vi "Change Settings.vi"(8 "error in (no error)":errorcluster) -> (0 "error out":errorcluster)   [LabVIEW 2023]
doc: "Presents an interface to change any settings that have been established in the application."
uses:
  CTLs/Hotkey Type.ctl
  <vilib>/Utility/config.llb/Config Data RefNum.ctl
  CTLs/Hotkey Values.ctl
  CTLs/FGV Actions.ctl
  2b057859-5186-41e9-9ab4-790756e7a186.vi
  a5ac09e5-38d3-43bc-9feb-68748838b8f7.vi
  <vilib>/Utility/inputDevices.llb/closeKeyboard.vi
  <vilib>/Utility/inputDevices.llb/keyboardAcquire.vi
  FaKI State Machine/FaKI State Machine.lvlib
  <vilib>/Utility/config.llb/NI_LVConfig.lvlib
panel:
  in  "Hotkey Type":T1
  in  "Start/Stop":bool
  in  "Exit":bool
  # "Change Hotkey\nPress Start Listening and hold down a key combination for five seconds to assign it as a hotkey."
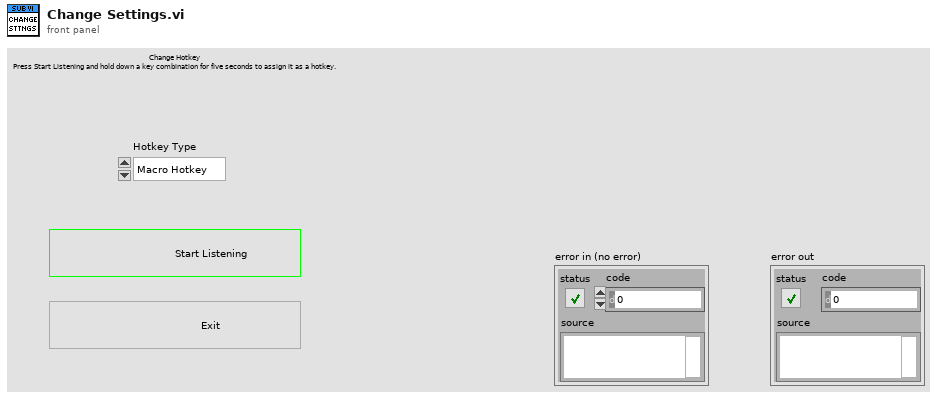
[diagram p1: front panel]
types:
  T1 = typedef "Hotkey Type.ctl" = enum16{"Macro Hotkey", "Abort Hotkey"}
  T2 = enum32{"Invalid", "Standard", "Closed", "Hidden", "Minimized", "Maximized"}
  T3 = enum32{"invalid app kind", "Development System", "Run Time System", "Student Edition", "Embedded LabVIEW", "Evaluation", "Custom"}
  T4 = typedef "FGV Actions.ctl" = enum16{"Read", "Write"}
  T5 = typedef "NI_LVConfig.lvlib/Config Data RefNum.ctl" = refnum<k1>
  T6 = typedef "Hotkey Values.ctl" = cluster{"Macro Hotkey":enum16{"0", "1", "2", "3", "4", "5", "6", "7", "8", "9", "A", "B", "C", "D", "E", "F", "G", "H", "I", "J", "K", "L", "M", "N", "O", "P", "Q", "R", "S", "T", "U", "V", "W", "X", "Y", "Z", "F1", "F2", "F3", "F4", "F5", "F6", "F7", "F8", "F9", "F10", "F11", "F12", "F13", "F14", "F15", "ADD", "BACK", "BACKSLASH", "CAPITAL", "COMMA", "DECIMAL", "DELETE", "DIVIDE", "DOWN", "END", "EQUALS", "ESCAPE", "GRAVE (`)", "HOME", "INSERT", "LBRACKET", "LCONTROL", "LEFT", "L ALT", "LSHIFT", "LWIN", "MINUS", "MULTIPLY", "NEXT", "NUMLOCK", "NUMPAD_0", "NUMPAD_1", "NUMPAD_2", "NUMPAD_3", "NUMPAD_4", "NUMPAD_5", "NUMPAD_6", "NUMPAD_7", "NUMPAD_8", "NUMPAD_9", "PAUSE", "PERIOD", "PRIOR (PG UP)", "RBRACKET", "RCONTROL", "RETURN", "RIGHT", "R ALT", "RSHIFT", "RWIN", "SCROLL", "SEMICOLON", "SLASH", "SPACE", "SUBTRACT", "TAB", "UP", "ENTER (num pad)", "' (quote)"}[], "Abort Hotkey":enum16{"0", "1", "2", "3", "4", "5", "6", "7", "8", "9", "A", "B", "C", "D", "E", "F", "G", "H", "I", "J", "K", "L", "M", "N", "O", "P", "Q", "R", "S", "T", "U", "V", "W", "X", "Y", "Z", "F1", "F2", "F3", "F4", "F5", "F6", "F7", "F8", "F9", "F10", "F11", "F12", "F13", "F14", "F15", "ADD", "BACK", "BACKSLASH", "CAPITAL", "COMMA", "DECIMAL", "DELETE", "DIVIDE", "DOWN", "END", "EQUALS", "ESCAPE", "GRAVE (`)", "HOME", "INSERT", "LBRACKET", "LCONTROL", "LEFT", "L ALT", "LSHIFT", "LWIN", "MINUS", "MULTIPLY", "NEXT", "NUMLOCK", "NUMPAD_0", "NUMPAD_1", "NUMPAD_2", "NUMPAD_3", "NUMPAD_4", "NUMPAD_5", "NUMPAD_6", "NUMPAD_7", "NUMPAD_8", "NUMPAD_9", "PAUSE", "PERIOD", "PRIOR (PG UP)", "RBRACKET", "RCONTROL", "RETURN", "RIGHT", "R ALT", "RSHIFT", "RWIN", "SCROLL", "SEMICOLON", "SLASH", "SPACE", "SUBTRACT", "TAB", "UP", "ENTER (num pad)", "' (quote)"}[]}
  T7 = cluster{"Core":cluster{"Current VI Reference":refnum<vi>, "Close Panel on Exit?":bool}, "Config":T5, "Keyboard":refnum<k1>, "Last":enum16{"0", "1", "2", "3", "4", "5", "6", "7", "8", "9", "A", "B", "C", "D", "E", "F", "G", "H", "I", "J", "K", "L", "M", "N", "O", "P", "Q", "R", "S", "T", "U", "V", "W", "X", "Y", "Z", "F1", "F2", "F3", "F4", "F5", "F6", "F7", "F8", "F9", "F10", "F11", "F12", "F13", "F14", "F15", "ADD", "BACK", "BACKSLASH", "CAPITAL", "COMMA", "DECIMAL", "DELETE", "DIVIDE", "DOWN", "END", "EQUALS", "ESCAPE", "GRAVE (`)", "HOME", "INSERT", "LBRACKET", "LCONTROL", "LEFT", "L ALT", "LSHIFT", "LWIN", "MINUS", "MULTIPLY", "NEXT", "NUMLOCK", "NUMPAD_0", "NUMPAD_1", "NUMPAD_2", "NUMPAD_3", "NUMPAD_4", "NUMPAD_5", "NUMPAD_6", "NUMPAD_7", "NUMPAD_8", "NUMPAD_9", "PAUSE", "PERIOD", "PRIOR (PG UP)", "RBRACKET", "RCONTROL", "RETURN", "RIGHT", "R ALT", "RSHIFT", "RWIN", "SCROLL", "SEMICOLON", "SLASH", "SPACE", "SUBTRACT", "TAB", "UP", "ENTER (num pad)", "' (quote)"}[], "Hotkeys":T6}
  T8 = enum16{"0", "1", "2", "3", "4", "5", "6", "7", "8", "9", "A", "B", "C", "D", "E", "F", "G", "H", "I", "J", "K", "L", "M", "N", "O", "P", "Q", "R", "S", "T", "U", "V", "W", "X", "Y", "Z", "F1", "F2", "F3", "F4", "F5", "F6", "F7", "F8", "F9", "F10", "F11", "F12", "F13", "F14", "F15", "ADD", "BACK", "BACKSLASH", "CAPITAL", "COMMA", "DECIMAL", "DELETE", "DIVIDE", "DOWN", "END", "EQUALS", "ESCAPE", "GRAVE (`)", "HOME", "INSERT", "LBRACKET", "LCONTROL", "LEFT", "L ALT", "LSHIFT", "LWIN", "MINUS", "MULTIPLY", "NEXT", "NUMLOCK", "NUMPAD_0", "NUMPAD_1", "NUMPAD_2", "NUMPAD_3", "NUMPAD_4", "NUMPAD_5", "NUMPAD_6", "NUMPAD_7", "NUMPAD_8", "NUMPAD_9", "PAUSE", "PERIOD", "PRIOR (PG UP)", "RBRACKET", "RCONTROL", "RETURN", "RIGHT", "R ALT", "RSHIFT", "RWIN", "SCROLL", "SEMICOLON", "SLASH", "SPACE", "SUBTRACT", "TAB", "UP", "ENTER (num pad)", "' (quote)"}[]
  T9 = cluster{"Current VI Reference":refnum<vi>, "Close Panel on Exit?":bool}
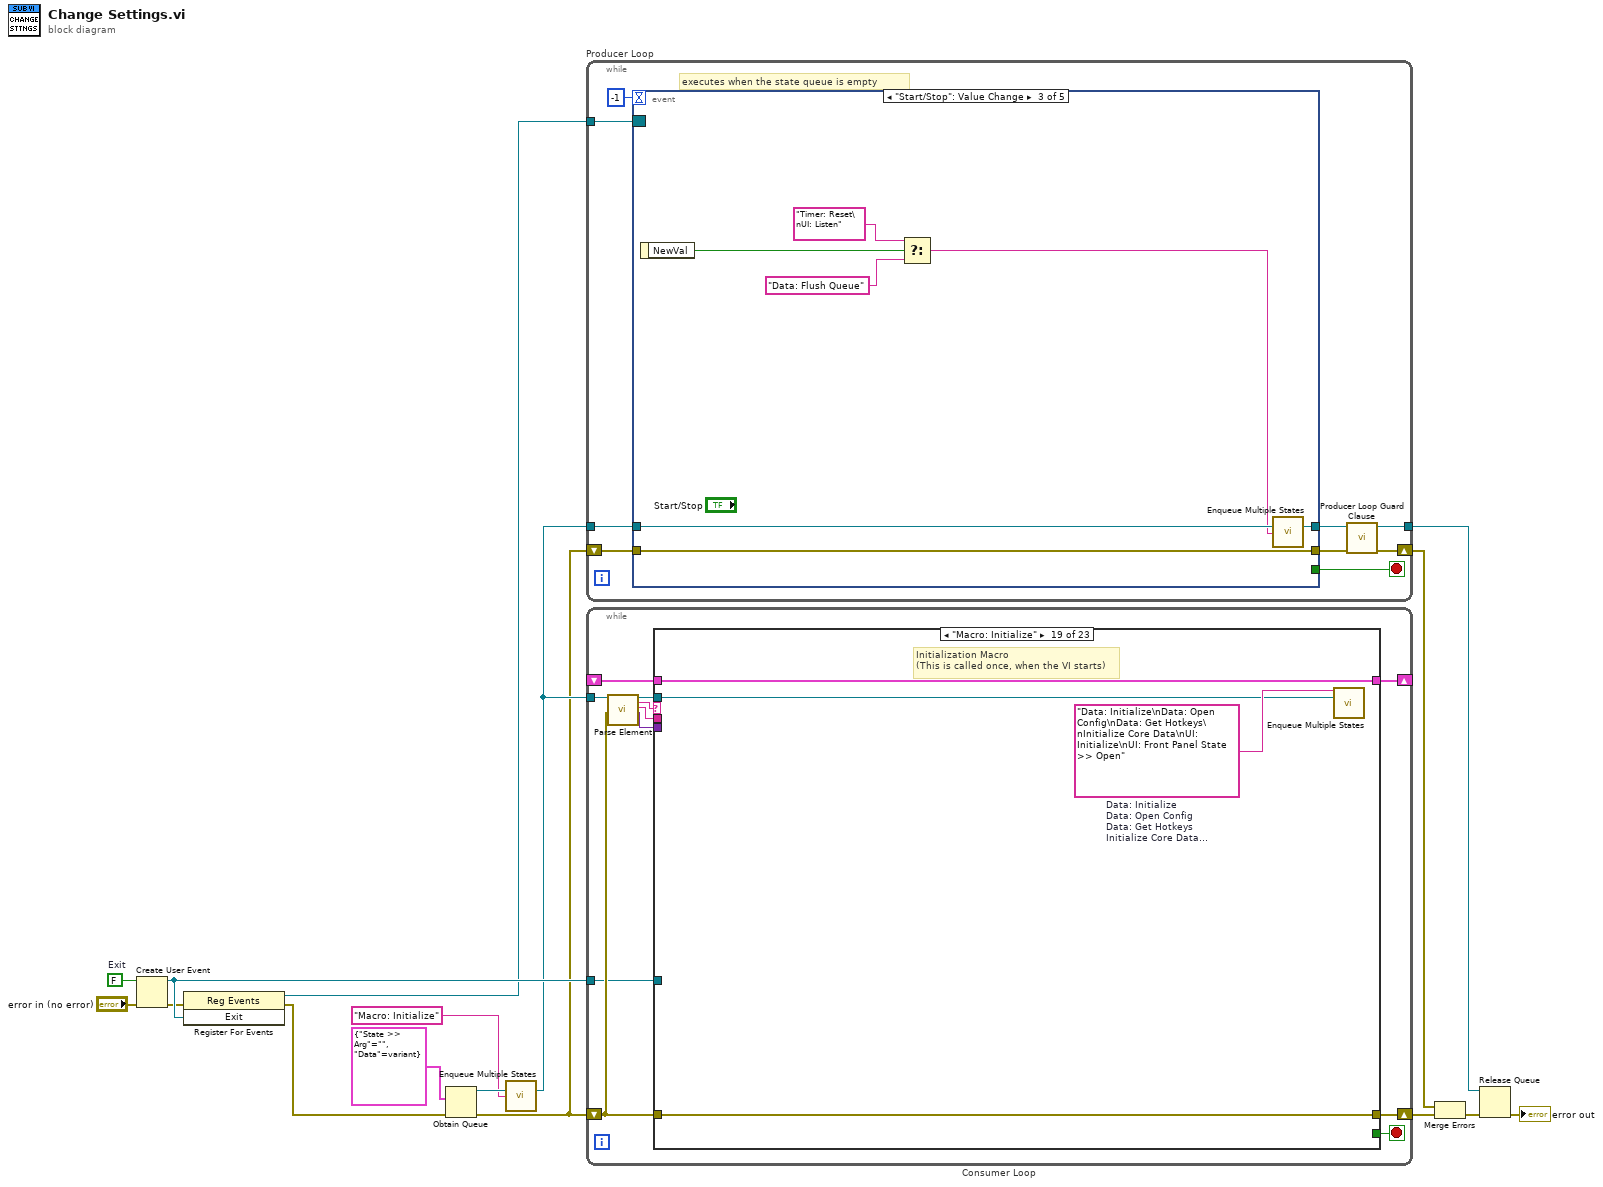
[diagram p0: block diagram]
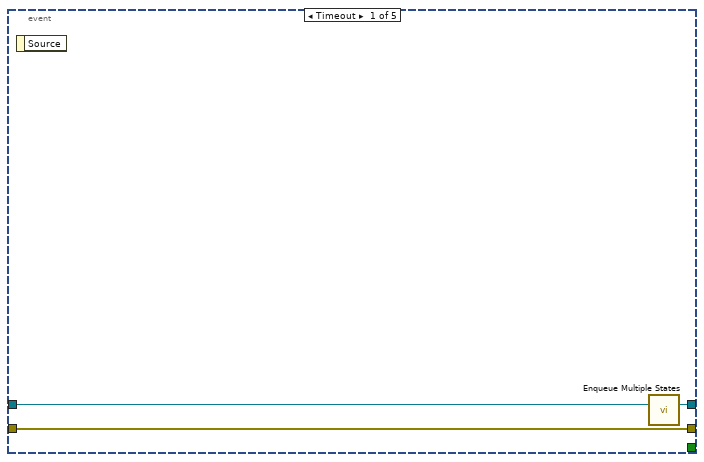
[diagram p2: hidden frame]
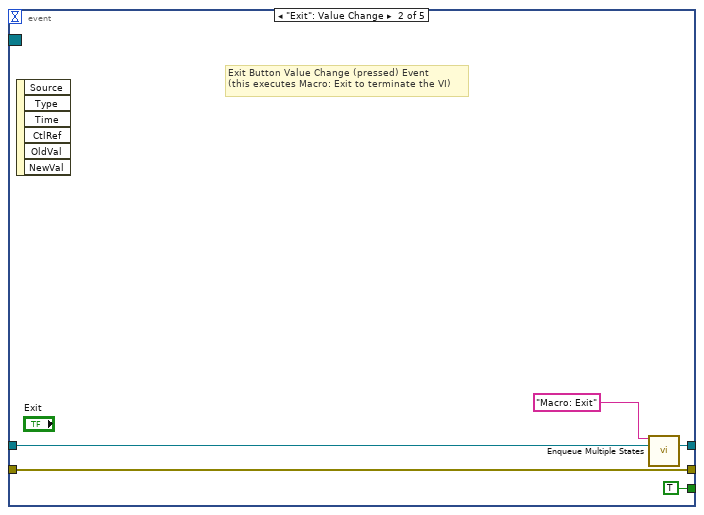
[diagram p3: hidden frame]
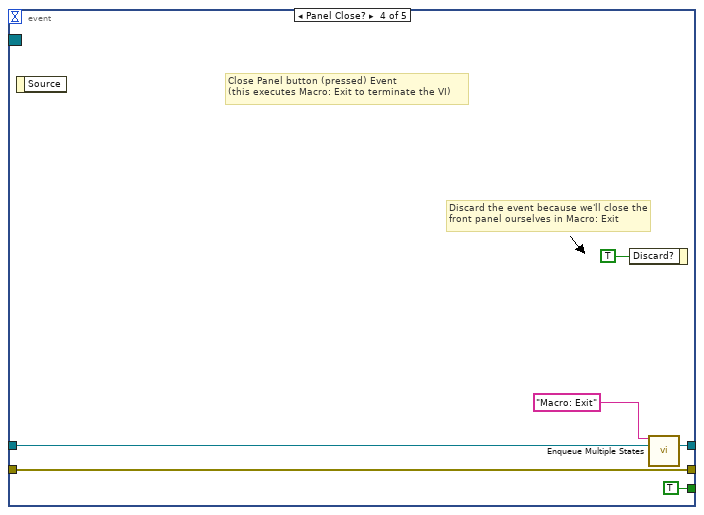
[diagram p4: hidden frame]
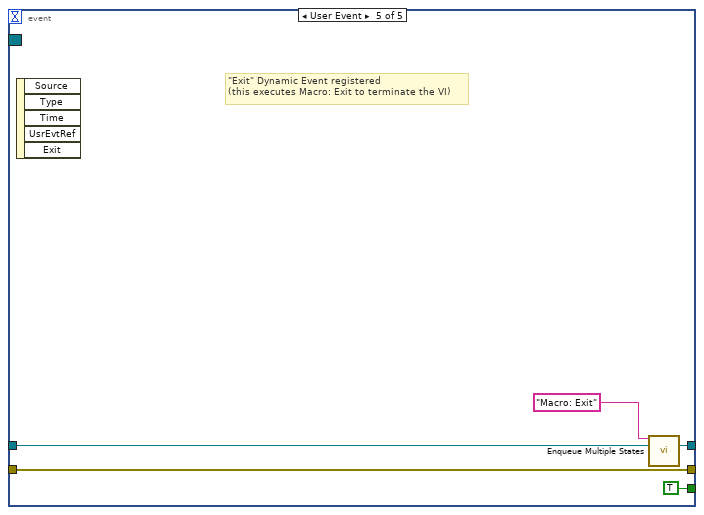
[diagram p5: hidden frame]
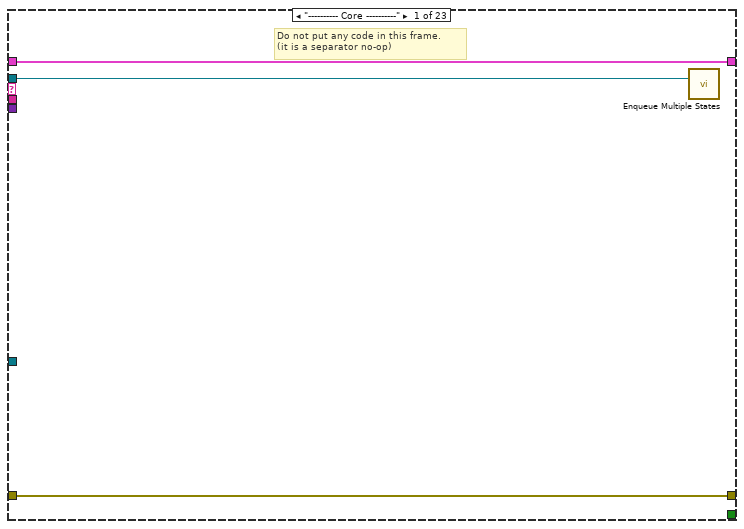
[diagram p6: hidden frame]
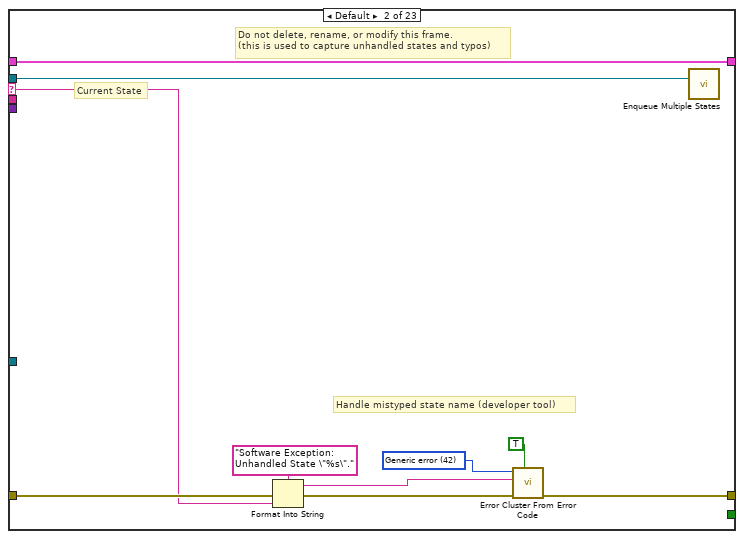
[diagram p7: hidden frame]
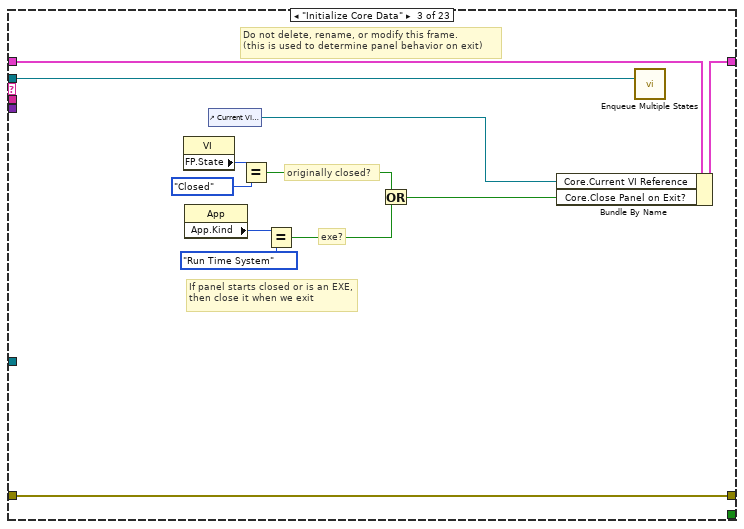
[diagram p8: hidden frame]
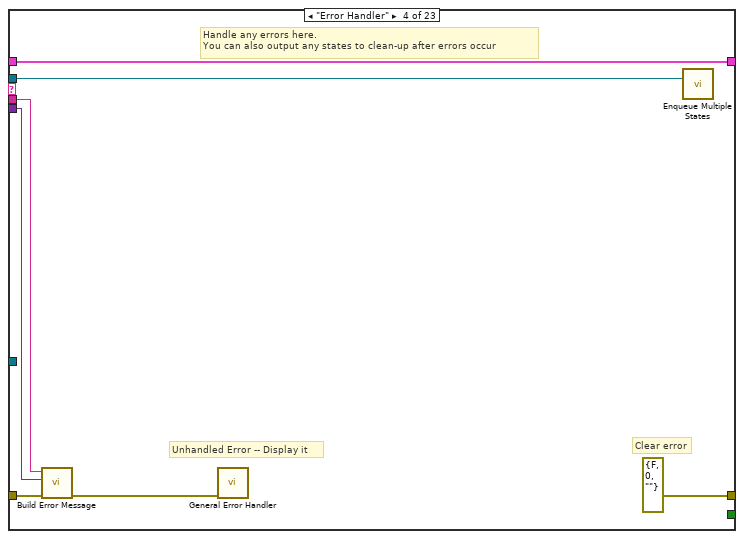
[diagram p9: hidden frame]
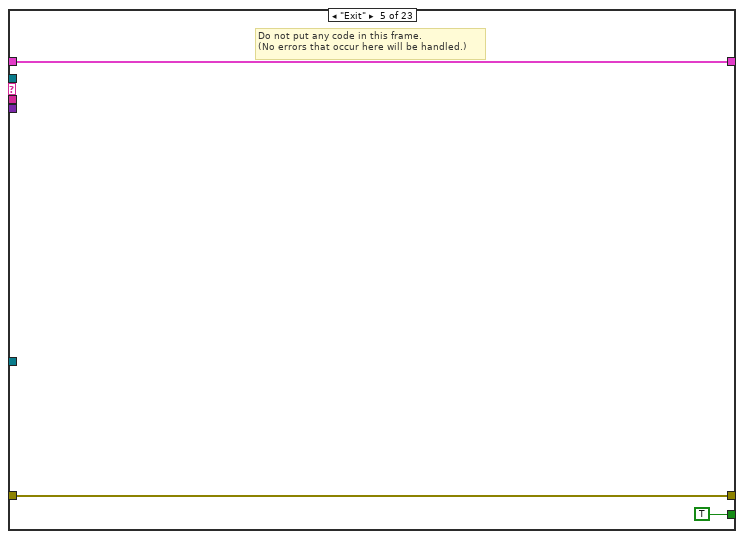
[diagram p10: hidden frame]
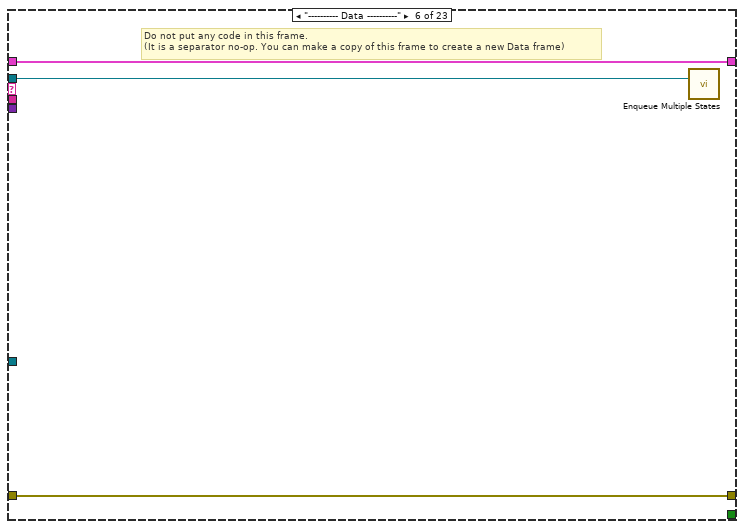
[diagram p11: hidden frame]
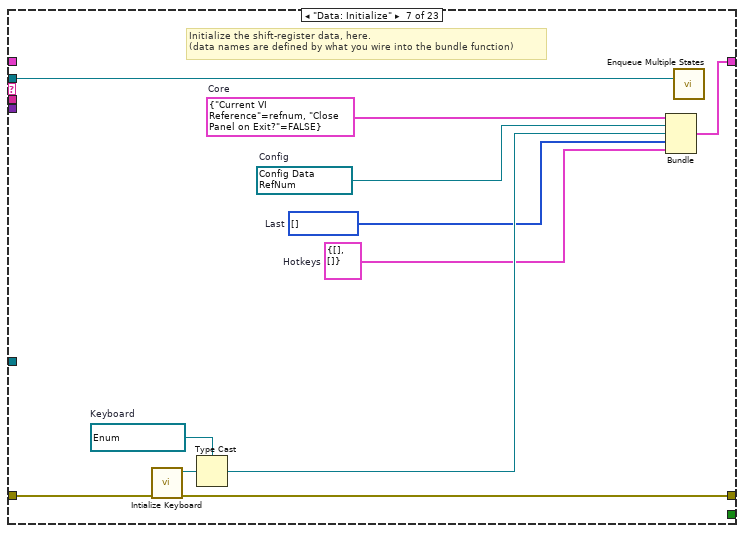
[diagram p12: hidden frame]
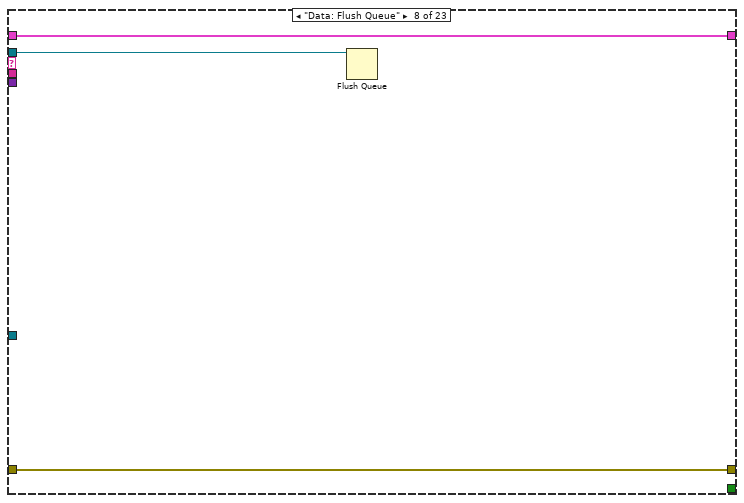
[diagram p13: hidden frame]
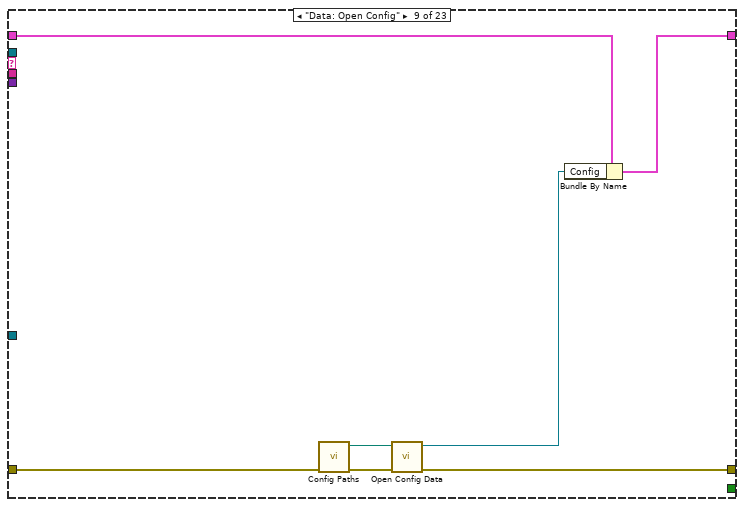
[diagram p14: hidden frame]
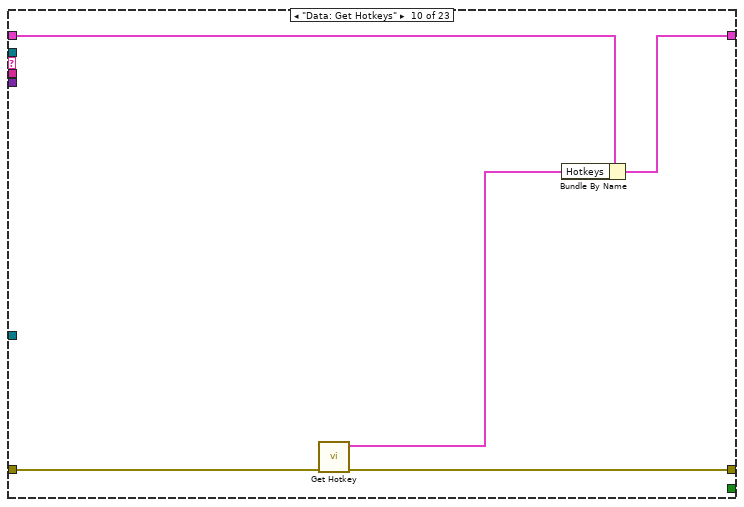
[diagram p15: hidden frame]
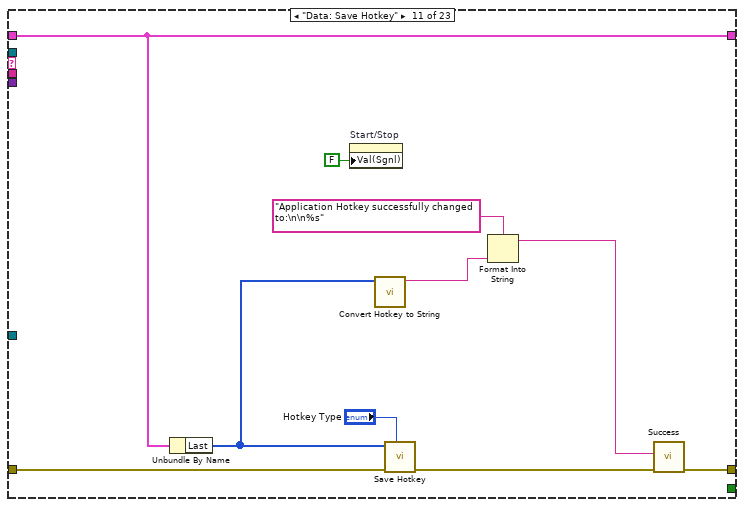
[diagram p16: hidden frame]
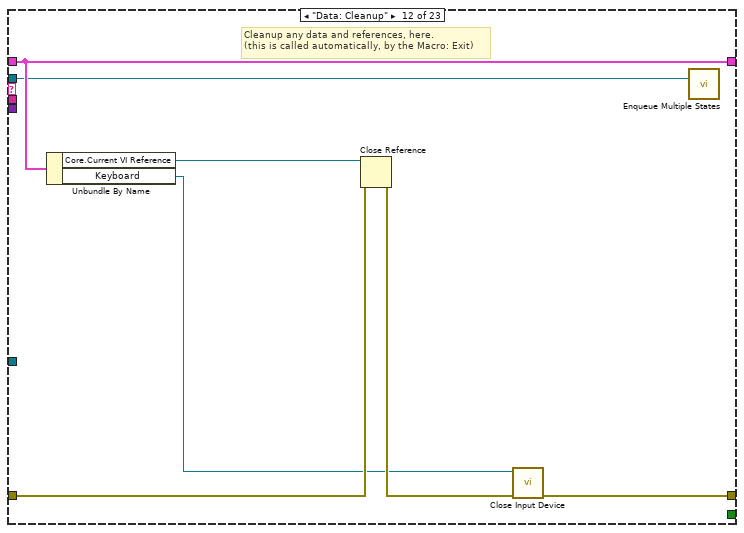
[diagram p17: hidden frame]
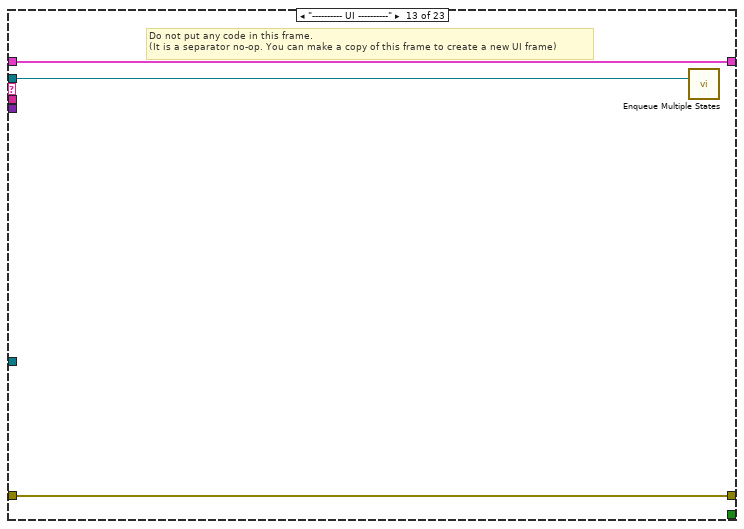
[diagram p18: hidden frame]
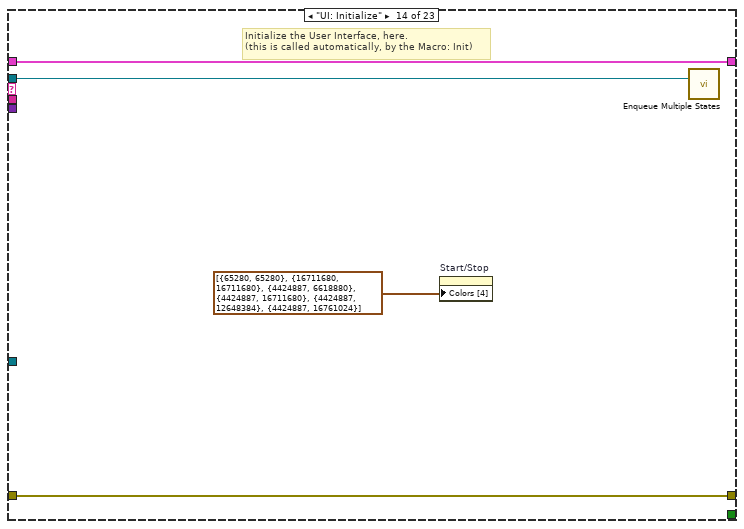
[diagram p19: hidden frame]
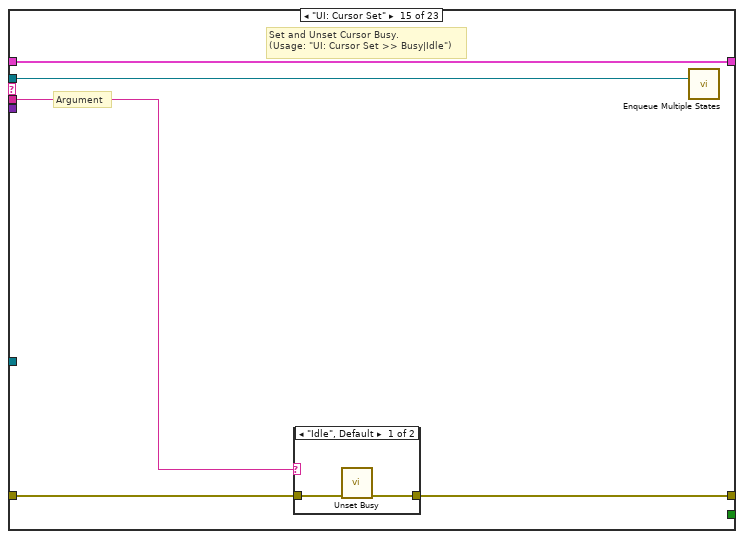
[diagram p20: hidden frame]
diagram:
  w13 = FALSE  # Exit
  n1 = Create User Event(user event datatype=w13, error in="error in (no error)") -> (user event=w16:refnum<user-event>, error out=w12:errorcluster)
  n2 = register-events(error in=w12, w16) -> (reference out=w15:refnum<event-registration>, error out=w14:errorcluster)  [unwired: 1 in]
  n3 = Obtain Queue(element data type=cluster{"State >> Arg":string, "Data":variant} {"State >> Arg"="", "Data"=variant}, error in (no error)=w14) -> (queue out=w6:refnum<queue>, error out=w3:errorcluster)  [unwired: 3 in, 1 out]
  n4 = call "Enqueue Multiple States.vi"("queue in"=w6, "State(s) at Back"="Macro: Initialize") -> ("queue out"=w7:refnum<queue>)  [unwired: 13 in]
  n5 = while "Producer Loop" {
    shift-right: [w20] -> w9
    shift-left: w3 -> [w25]
    tunnel: w15 -> [w17]
    tunnel: w7 -> [w23]
    tunnel: [w18] -> w11
    stop <- w22 stop-if-true
    # "executes when the state queue is empty"
    n6 = event shown="[2] \"Start/Stop\": Value Change" {
      selector: w17 -> [_ _ _ _ _]
      dyn-events: _ -> [_ _ _ _ _]
      timeout: -1 ("Timeout") -> [_ _ _ _ _]
      tunnel: [w26 w33 w40 w46 w51] -> w21
      tunnel: w25 -> [w26 w33 w40 w46 w51]
      tunnel: w23 -> [w27 w32 w39 w43 w49]
      tunnel: [w28 w30 w38 w42 w48] -> w19
      tunnel: [_ TRUE _ TRUE TRUE] -> w22
      event Timeout {
        n7 = event-data() -> ()  [unwired: 1 in, 1 out]
        n8 = call "Enqueue Multiple States.vi"("queue in"=w27) -> ("queue out"=w28:refnum<queue>)  [unwired: 14 in]
      }
      event "Exit": Value Change {
        # "Exit Button Value Change (pressed) Event\n(this executes Macro: Exit to terminate the VI)"
        n9 = event-data() -> ()  [unwired: 1 in, 6 out]
        n10 = call "Enqueue Multiple States.vi"("State(s) at Front"="Macro: Exit", "queue in"=w32) -> ("queue out"=w30:refnum<queue>)  [unwired: 13 in]
      }
      event "Start/Stop": Value Change {
        n11 = event-data() -> ("NewVal"=w37:bool)  [unwired: 1 in]
        n12 = Select(t="Timer: Reset\nUI: Listen", s=w37, f="Data: Flush Queue") -> (s? t:f=w34:string)
        n13 = call "Enqueue Multiple States.vi"("queue in"=w39, "State(s) at Back"=w34) -> ("queue out"=w38:refnum<queue>)  [unwired: 13 in]
      }
      event Panel Close? {
        # "Discard the event because we'll close the front panel ourselves in Macro: Exit"
        # "Close Panel button (pressed) Event\n(this executes Macro: Exit to terminate the VI)"
        n14 = event-data() -> ()  [unwired: 1 in, 1 out]
        n15 = event-data("Discard?"=TRUE) -> ()  [unwired: 1 in, 1 out]
        n16 = call "Enqueue Multiple States.vi"("State(s) at Front"="Macro: Exit", "queue in"=w43) -> ("queue out"=w42:refnum<queue>)  [unwired: 13 in]
      }
      event User Event {
        # "\"Exit\" Dynamic Event registered\n(this executes Macro: Exit to terminate the VI)"
        n17 = event-data() -> ()  [unwired: 1 in, 5 out]
        n18 = call "Enqueue Multiple States.vi"("State(s) at Front"="Macro: Exit", "queue in"=w49) -> ("queue out"=w48:refnum<queue>)  [unwired: 13 in]
      }
    }
    n19 = call "Producer Loop Guard Clause.vi"("error in (no error)"=w21, "queue in"=w19) -> ("error out"=w20:errorcluster, "queue out"=w18:refnum<queue>)  [unwired: 8 in]
  }
  n20 = while "Consumer Loop" {
    shift-right: [w59] -> _
    shift-left: _ -> [w58]
    shift-right: [w62] -> w8
    shift-left: w3 -> [w61]
    tunnel: w7 -> [w57]
    tunnel: w16 -> [w52]
    stop <- w60 stop-if-true
    n21 = call "Parse Element.vi"("queue in"=w57, "error in (no error)"=w61) -> ("queue out"=w56:refnum<queue>, "State"=w55:string, "Arg"=w54:string, "Data"=w53:variant)  [unwired: 14 in]
    n22 = case shown="\"Macro: Initialize\"" w55 {
      selector: w55 -> [_ w67 _ _ _ _ _ _ _ _ _ _ _ _ _ _ _ _ _ _ _ _ _]
      tunnel: w56 -> [w63 w66 w76 w92 _ w98 w109 w114 _ _ _ w140 w144 w148 w151 w160 w243 w266 w269 w276 w282 _ w291]
      tunnel: w54 -> [_ _ _ w88 _ _ _ _ _ _ _ _ _ _ w152 w161 _ _ _ _ _ _ _]
      tunnel: w58 -> [w64 w69 w82 w93 w96 w99 _ w113 w118 w125 w127 w141 w145 w149 w153 w163 w242 w267 w271 w280 w283 w289 w298]
      tunnel: [w65 w74 w87 errorcluster {"status"=FALSE, "code"=0, "source"=""} ("error out") w97 w100 w103 w112 w119 w123 w134 w138 w146 w150 w154 w164 w251 w268 w272 w281 w284 w287 w296] -> w62
      tunnel: w61 -> [w65 w73 w87 w91 w97 w100 w106 w112 w120 w126 w132 w143 w146 w150 w155 w165 w252 w268 w272 w281 w284 w288 w297]
      tunnel: [_ _ _ _ TRUE _ _ _ _ _ _ _ _ _ _ _ _ _ _ _ _ _ _] -> w60
      tunnel: [w64 w69 w86 w93 w96 w99 w111 w113 w117 w124 w127 w141 w145 w149 w153 w163 w241 w267 w271 w280 w283 w289 w298] -> w59
      tunnel: w53 -> [_ _ _ w89 _ _ _ _ _ _ _ _ _ _ _ _ _ _ _ _ _ _ _]
      tunnel: w52 -> [_ _ _ _ _ _ _ _ _ _ _ _ _ _ _ _ _ _ _ _ _ _ _]
      frame "---------- Core ----------" {
        # "Do not put any code in this frame.\n(it is a separator no-op)"
        n23 = call "Enqueue Multiple States.vi"("queue in"=w63) -> ()  [unwired: 14 in, 1 out]
      }
      frame Default {
        w71 = 42 items=["No error", "Argument error", "Memory is full", "Out of zone", "End of file", "File already open", "Generic file I/O error", "File not found", "File permission error", "Disk is full", "Duplicate path", "Too many files open", "System feature not enabled", "Resource file not found", "Cannot add resource", "Resource not found", "Image not found", "Image memory error", "Pen does not exist", "Config type invalid", "Config token not found", "Config parse error", "Config memory error", "Bad external code format", "Bad external code offset", "External code not present", "Null window", "Destroy window error", "Null menu", "Print aborted", "Bad print record", "Print driver error", "Windows error during printing", "Memory error during printing", "Print dialog error", "Generic print error", "Invalid device refnum", "Device not found", "Device parameter error", "Device unit error", "Cannot open device", "Device call aborted", "Generic error", "Cancelled by user", "Object ID too low", "Object ID too high", "Object not in heap", "Unknown heap", "Unknown object (invalid DefProc)", "Unknown object (DefProc not in table)", "Message out of range", "Invalid (null) method", "Unknown message", "Manager call not supported", "Bad address", "Network operation in progress", "Network operation timed out", "Connection is busy", "Network attribute not supported", "Network error", "Address in use", "System out of memory", "Connection aborted", "Connection refused", "Not connected", "Already connected", "Connection closed", "Initialization error (interapplication manager)", "Bad occurrence", "Wait on unbound occurrence handler", "Occurrence queue overflow", "Datalog type conflict", "Unused", "Unrecognized type (interapplication manager)", "Memory corrupt", "Failed to make temporary DLL", "Old CIN version", "Drag socket not found", "Failed to load drop-object", "Failed to register OLE object", "Failed to release OLE object", "Format specifier type mismatch", "Unknown format specifier", "Too few format specifiers", "Too many format specifiers", "Scan failed", "Newer CIN version", "Error converting to variant", "Runtime menu error", "Password tampered", "Variant attribute not found", "Incompatible variant data type", "Event data is not available", "Event Store is not present", "Occurrence is not found", "Event Queue is not created", "Event info is not available", "Refnum passed is NULL", "Error retrieving Class GUID", "Error retrieving CoClass GUID", "Error retrieving TypeLib GUID.", "Bad built application magic bytes.", "Specific driver is different from the specific driver associated with the Logical Name.", "There is no session opened to the class driver.", "Max Error", "MAX - Error with config objects", "MAX - Error loading configuration", "MAX - Group not supported"]
        # "Current State"
        # "Do not delete, rename, or modify this frame.\n(this is used to capture unhandled states and typos)"
        # "Handle mistyped state name (developer tool)"
        n24 = Format Into String(format string="Software Exception: Unhandled State \"%s\"." ("message"), error in=w73, w67) -> (resulting string=w70:string, error out=w75:errorcluster)  [unwired: 1 in]
        n25 = call <vilib>:"Error Cluster From Error Code.vi"("show call chain? (False)"=TRUE, "error in (no error)"=w75, "error message (\"\")"=w70, "error code (0)"=w71) -> ("error out"=w74:errorcluster)  [unwired: 5 in]
        n26 = call "Enqueue Multiple States.vi"("queue in"=w66) -> ()  [unwired: 14 in, 1 out]
      }
      frame "Initialize Core Data" {
        # "Do not delete, rename, or modify this frame.\n(this is used to determine panel behavior on exit)"
        # "originally closed?"
        # "exe?"
        # "If panel starts closed or is an EXE, then close it when we exit"
        n27 = property class="VI"() -> ("FP.State"=w79:T2)  [unwired: 2 in, 2 out]
        n28 = property class="App"() -> ("App.Kind"=w85:T3)  [unwired: 2 in, 2 out]
        n29 = control-ref of="Current VI Reference"() -> (w80:refnum<vi>)
        n30 = Equal?(x=w79, y=T2."Closed" ("Front Panel Window:State")) -> (x = y?=w77:bool)
        n31 = Equal?(x=w85, y=T3."Run Time System" ("Application:Kind")) -> (x = y?=w83:bool)
        n32 = Or(x=w77, y=w83) -> (x .or. y?=w81:bool)
        n33 = Bundle By Name(cluster=w82, "Core.Current VI Reference"=w80, "Core.Close Panel on Exit?"=w81) -> (w86:T7)
        n34 = call "Enqueue Multiple States.vi"("queue in"=w76) -> ()  [unwired: 14 in, 1 out]
      }
      frame "Error Handler" {
        # "Unhandled Error -- Display it"
        # "Handle any errors here.\nYou can also output any states to clean-up after errors occur"
        # "Clear error"
        n35 = call "Build Error Message.vi"("error in (no error)"=w91, "Data"=w89, "Arg"=w88) -> ("error out"=w90:errorcluster)  [unwired: 8 in]
        n36 = call <vilib>:"General Error Handler.vi"("error in (no error)"=w90) -> ()  [unwired: 10 in, 5 out]
        n37 = call "Enqueue Multiple States.vi"("queue in"=w92) -> ()  [unwired: 14 in, 1 out]
      }
      frame "Exit" {
        # "Do not put any code in this frame.\n(No errors that occur here will be handled.)"
      }
      frame "---------- Data ----------" {
        # "Do not put any code in this frame.\n(It is a separator no-op. You can make a copy of this frame to create a new Data frame)"
        n38 = call "Enqueue Multiple States.vi"("queue in"=w98) -> ()  [unwired: 14 in, 1 out]
      }
      frame "Data: Initialize" {
        w101 = T6 {"Macro Hotkey"=[], "Abort Hotkey"=[]}  # Hotkeys
        w102 = T8 [] items=["0", "1", "2", "3", "4", "5", "6", "7", "8", "9", "A", "B", "C", "D", "E", "F", "G", "H", "I", "J", "K", "L", "M", "N", "O", "P", "Q", "R", "S", "T", "U", "V", "W", "X", "Y", "Z", "F1", "F2", "F3", "F4", "F5", "F6", "F7", "F8", "F9", "F10", "F11", "F12", "F13", "F14", "F15", "ADD", "BACK", "BACKSLASH", "CAPITAL", "COMMA", "DECIMAL", "DELETE", "DIVIDE", "DOWN", "END", "EQUALS", "ESCAPE", "GRAVE (`)", "HOME", "INSERT", "LBRACKET", "LCONTROL", "LEFT", "L ALT", "LSHIFT", "LWIN", "MINUS", "MULTIPLY", "NEXT", "NUMLOCK", "NUMPAD_0", "NUMPAD_1", "NUMPAD_2", "NUMPAD_3", "NUMPAD_4", "NUMPAD_5", "NUMPAD_6", "NUMPAD_7", "NUMPAD_8", "NUMPAD_9", "PAUSE", "PERIOD", "PRIOR (PG UP)", "RBRACKET", "RCONTROL", "RETURN", "RIGHT", "R ALT", "RSHIFT", "RWIN", "SCROLL", "SEMICOLON", "SLASH", "SPACE", "SUBTRACT", "TAB", "UP", "ENTER (num pad)", "' (quote)"]  # Last
        w105 = T5 refnum items=["config data"]  # Config
        w107 = refnum<k1> refnum items=["KEYBOARD"]  # Keyboard
        w110 = T9 {"Current VI Reference"=refnum, "Close Panel on Exit?"=FALSE}  # Core
        # "Initialize the shift-register data, here.\n(data names are defined by what you wire into the bundle function)"
        n39 = call <vilib>:"Intialize Keyboard.vi"("error in (no error)"=w106) -> ("error out"=w103:errorcluster, "device ID"=w108:refnum<k1>)  [unwired: 9 in]
        n40 = Type Cast(type=w107, x=w108) -> (*(type *) &x=w104:refnum<k1>)
        n41 = Bundle("Core"=w110, "Config"=w105, "Keyboard"=w104, "Last"=w102, "Hotkeys"=w101) -> (w111:T7)  [unwired: 1 in]
        n42 = call "Enqueue Multiple States.vi"("queue in"=w109) -> ()  [unwired: 14 in, 1 out]
      }
      frame "Data: Flush Queue" {
        n43 = Flush Queue(queue=w114) -> ()  [unwired: 1 in, 3 out]
      }
      frame "Data: Open Config" {
        n44 = call "Config Paths.vi"("error in (no error)"=w120) -> ("error out"=w121:errorcluster, "Global Config"=w115:path)  [unwired: 8 in, 1 out]
        n45 = call <vilib>:"Open Config Data.vi"("error in (no error)"=w121, "configuration file path"=w115) -> ("error out"=w119:errorcluster, "refnum"=w116:T5)  [unwired: 7 in, 1 out]
        n46 = Bundle By Name(cluster=w118, "Config"=w116) -> (w117:T7)
      }
      frame "Data: Get Hotkeys" {
        n47 = call "Get Hotkey.vi"("error in (no error)"=w126) -> ("error out"=w123:errorcluster, "Hotkey Values"=w122:T6)  [unwired: 9 in]
        n48 = Bundle By Name(cluster=w125, "Hotkeys"=w122) -> (w124:T7)
      }
      frame "Data: Save Hotkey" {
        n49 = Unbundle By Name(w127) -> ("Last"=w129:T8)
        n50 = property on="Start/Stop" class="Bool (strict)"("Val(Sgnl)"=FALSE ("Value (Signaling)")) -> ()  [unwired: 2 in, 2 out]
        n51 = call "Convert Hotkey to String.vi"("Hotkey"=w129) -> ("String"=w128:string)  [unwired: 10 in]
        n52 = call "Save Hotkey.vi"("Hotkey Type"="Hotkey Type", "error in (no error)"=w132, "Hotkey"=w129) -> ("error out"=w131:errorcluster)  [unwired: 8 in]
        n53 = Format Into String(format string="Application Hotkey successfully changed to:\n\n%s", w128) -> (resulting string=w135:string)  [unwired: 2 in, 1 out]
        n54 = call "Success"("error in (no error)"=w131, "Message"=w135) -> ("error out"=w134:errorcluster)  [unwired: 8 in, 1 out]
      }
      frame "Data: Cleanup" {
        # "Cleanup any data and references, here.\n(this is called automatically, by the Macro: Exit)"
        n55 = Unbundle By Name(w141) -> ("Core.Current VI Reference"=w142:refnum<vi>, "Keyboard"=w137:refnum<k1>)
        n56 = Close Reference(reference=w142, error in (no error)=w143) -> (error out=w139:errorcluster)
        n57 = call-poly <vilib>:"Close Input Device.vi"("error in (no error)"=w139, "device ID"=w137) -> ("error out"=w138:errorcluster)  [unwired: 8 in]
        n58 = call "Enqueue Multiple States.vi"("queue in"=w140) -> ()  [unwired: 14 in, 1 out]
      }
      frame "---------- UI ----------" {
        # "Do not put any code in this frame.\n(It is a separator no-op. You can make a copy of this frame to create a new UI frame)"
        n59 = call "Enqueue Multiple States.vi"("queue in"=w144) -> ()  [unwired: 14 in, 1 out]
      }
      frame "UI: Initialize" {
        # "Initialize the User Interface, here.\n(this is called automatically, by the Macro: Init)"
        n60 = property on="Start/Stop" class="Bool (strict)"("Colors [4]"=cluster{u32, u32}[] [{65280, 65280}, {16711680, 16711680}, {4424887, 6618880}, {4424887, 16711680}, {4424887, 12648384}, {4424887, 16761024}]) -> ()  [unwired: 2 in, 2 out]
        n61 = call "Enqueue Multiple States.vi"("queue in"=w148) -> ()  [unwired: 14 in, 1 out]
      }
      frame "UI: Cursor Set" {
        # "Argument"
        # "Set and Unset Cursor Busy.\n(Usage: \"UI: Cursor Set >> Busy|Idle\")"
        n62 = case shown="\"Idle\", Default" w152 {
          tunnel: w155 -> [w157 w159]
          tunnel: [w156 w158] -> w154
          frame "Idle", Default {
            n63 = call <vilib>:"Unset Busy.vi"("error in (no error)"=w157) -> ("error out"=w156:errorcluster)  [unwired: 10 in]
          }
          frame "Busy" {
            n64 = call <vilib>:"Set Busy.vi"("error in (no error)"=w159) -> ("error out"=w158:errorcluster)  [unwired: 9 in, 1 out]
          }
        }
        n65 = call "Enqueue Multiple States.vi"("queue in"=w151) -> ()  [unwired: 14 in, 1 out]
      }
      frame "UI: Front Panel State" {
        # "Argument"
        # "Set Front Panel Open or Closed\n(Usage: \"UI: Front Panel State >> Open|Close\")"
        n66 = Unbundle By Name(w163) -> ("Core.Current VI Reference"=w162:refnum<vi>)
        n67 = case shown="\"Open\", \"Standard\", Default" w161 {
          tunnel: w165 -> [w172 w186 w198 w211 w224]
          tunnel: [w173 w187 w199 w212 w225] -> w164
          tunnel: w162 -> [w170 w184 w196 w209 w222]
          frame "Open", "Standard", Default {
            w166 = T2."Standard" ("State")
            n68 = property class="VI"(reference=w170, error in=w172) -> (reference out=w169:refnum<vi>, error out=w171:errorcluster, "FP.State"=w168:T2)
            n69 = Not Equal?(x=w168, y=w166) -> (x != y?=w167:bool)
            n70 = case shown="True" w167 {
              tunnel: [w178 w179] -> w173
              tunnel: w171 -> [w177 w179]
              tunnel: w169 -> [w175 _]
              tunnel: w166 -> [w174 _]
              frame True {
                n71 = invoke class="VI" method="FP.Open"(reference=w175, error in=w177, "Activate"=TRUE, "State"=w174) -> (error out=w178:errorcluster)  [unwired: 1 in, 4 out]
              }
              frame False {
              }
            }
          }
          frame "Close", "Closed" {
            n72 = property class="VI"(reference=w184, error in=w186) -> (reference out=w183:refnum<vi>, error out=w185:errorcluster, "FP.State"=w181:T2)
            n73 = Not Equal?(x=w181, y=T2."Closed" ("Front Panel Window:State")) -> (x != y?=w180:bool)
            n74 = case shown="True" w180 {
              tunnel: [w188 w191] -> w187
              tunnel: w185 -> [w188 w190]
              tunnel: w183 -> [_ w189]
              frame False {
              }
              frame True {
                n75 = invoke class="VI" method="FP.Close"(reference=w189, error in=w190) -> (error out=w191:errorcluster)  [unwired: 1 in, 2 out]
              }
            }
          }
          frame "Hidden", "Hide" {
            w192 = T2."Hidden" ("State")
            n76 = property class="VI"(reference=w196, error in=w198) -> (reference out=w195:refnum<vi>, error out=w197:errorcluster, "FP.State"=w194:T2)
            n77 = Not Equal?(x=w194, y=w192) -> (x != y?=w193:bool)
            n78 = case shown="True" w193 {
              tunnel: [w203 w204] -> w199
              tunnel: w197 -> [w202 w204]
              tunnel: w195 -> [w201 _]
              tunnel: w192 -> [w200 _]
              frame True {
                n79 = invoke class="VI" method="FP.Open"(reference=w201, error in=w202, "State"=w200) -> (error out=w203:errorcluster)  [unwired: 2 in, 4 out]
              }
              frame False {
              }
            }
          }
          frame "Minimize", "Minimized" {
            w205 = T2."Minimized" ("State")
            n80 = property class="VI"(reference=w209, error in=w211) -> (reference out=w208:refnum<vi>, error out=w210:errorcluster, "FP.State"=w207:T2)
            n81 = Not Equal?(x=w207, y=w205) -> (x != y?=w206:bool)
            n82 = case shown="True" w206 {
              tunnel: [w216 w217] -> w212
              tunnel: w210 -> [w215 w217]
              tunnel: w208 -> [w214 _]
              tunnel: w205 -> [w213 _]
              frame True {
                n83 = invoke class="VI" method="FP.Open"(reference=w214, error in=w215, "State"=w213) -> (error out=w216:errorcluster)  [unwired: 2 in, 4 out]
              }
              frame False {
              }
            }
          }
          frame "Maximize", "Maximized" {
            w218 = T2."Maximized" ("State")
            n84 = property class="VI"(reference=w222, error in=w224) -> (reference out=w221:refnum<vi>, error out=w223:errorcluster, "FP.State"=w220:T2)
            n85 = Not Equal?(x=w220, y=w218) -> (x != y?=w219:bool)
            n86 = case shown="True" w219 {
              tunnel: [w229 w230] -> w225
              tunnel: w223 -> [w228 w230]
              tunnel: w221 -> [w227 _]
              tunnel: w218 -> [w226 _]
              frame True {
                n87 = invoke class="VI" method="FP.Open"(reference=w227, error in=w228, "State"=w226) -> (error out=w229:errorcluster)  [unwired: 2 in, 4 out]
              }
              frame False {
              }
            }
          }
        }
        n88 = call "Enqueue Multiple States.vi"("queue in"=w160) -> ()  [unwired: 14 in, 1 out]
      }
      frame "UI: Listen" {
        n89 = Unbundle By Name(w242) -> ("Hotkeys"=w237:T6, "Last"=w249:T8, "Keyboard"=w256:refnum<k1>)
        n90 = call "Stall Data Flow.vim"("value in"=w256, "milliseconds to wait"=u32 1) -> ("value out"=w254:refnum<k1>)  [unwired: 1 out]
        n91 = Empty Array?(array=w249) -> (empty?=w250:bool)
        n92 = call-poly <vilib>:"Acquire Input Data.vi"("device ID"=w254, "error in (no error)"=w252) -> ("keys pressed"=w255:T8, "error out"=w251:errorcluster)  [unwired: 15 in, 1 out]
        n93 = call "Enum to Array of Enums.vim"("enum"=Hotkey_Type."Macro Hotkey" ("Hotkey Type")) -> ("array of enums"=w239:T1[])
        n94 = Not(x=w250) -> (.not. x?=w247:bool)
        n95 = Sort 1D Array(array=w255) -> (sorted array=w236:T8)
        n96 = Equal?(x=w249, y=w236) -> (x = y?=w248:bool)
        n97 = for {
          tunnel: w239 -> [w260] mode=indexing
          tunnel: w237 -> [w261]
          tunnel: [w260] -> w234 if=w257
          tunnel: w236 -> [w259]
          tunnel: [w257] -> w232
          stop <- w257 stop-if-true
          n98 = case shown="\"Abort Hotkey\"" w260 {
            tunnel: w261 -> [w263 w265]
            tunnel: [w262 w264] -> w258
            frame "Macro Hotkey", Default {
              n99 = Unbundle By Name(w263) -> ("Macro Hotkey"=w262:T8)
            }
            frame "Abort Hotkey" {
              n100 = Unbundle By Name(w265) -> ("Abort Hotkey"=w264:T8)
            }
          }
          n101 = Equal?(x=w258, y=w259) -> (x = y?=w257:bool)
        }
        n102 = Not(x=w232) -> (.not. x?=w231:bool)
        n103 = Format Into String(format string="That key combination is already assigned as the %s.", w234) -> (resulting string=w233:string)  [unwired: 2 in, 1 out]
        n104 = Compound Arithmetic op=AND(w231, w247, w248) -> (w246:bool)
        n105 = call "Already Assigned"("Enable"=w232, "Message"=w233) -> ()  [unwired: 8 in, 2 out]
        n106 = Select(t="Timer: Poll", s=w246, f="Timer: Reset\nUI: Listen") -> (s? t:f=w240:string)
        n107 = call "Enqueue Multiple States.vi"("queue in"=w243, "State(s) at Back"=w240) -> ()  [unwired: 13 in, 1 out]
        n108 = Bundle By Name(cluster=w242, "Last"=w236) -> (w241:T7)
      }
      frame "---------- Macro ----------" {
        # "Do not put any code in this frame.\n(It is a separator no-op. You can make a copy of this frame to create a new Macro frame)"
        n109 = call "Enqueue Multiple States.vi"("queue in"=w266) -> ()  [unwired: 14 in, 1 out]
      }
      frame "Macro: Initialize" {
        w270 = "Data: Initialize\nData: Open Config\nData: Get Hotkeys\nInitialize Core Data\nUI: Initialize\nUI: Front Panel State >> Open"  # Data: Initialize Data: Open Config Data: Get Hotkeys Initialize Core Data UI: Initialize UI: Front Panel State >> Open
        # "Initialization Macro\n(This is called once, when the VI starts)"
        n110 = call "Enqueue Multiple States.vi"("State(s) at Front"=w270, "queue in"=w269) -> ()  [unwired: 13 in, 1 out]
      }
      frame "Macro: Exit" {
        # "Exit Macro\n(This is called once, when the VI exits)"
        n111 = Unbundle By Name(w280) -> ("Core.Close Panel on Exit?"=w279:bool)
        n112 = Select(t="UI: Front Panel State >> Close\n", s=w279, f="") -> (s? t:f=w275:string)
        n113 = Concatenate Strings(w275, "Data: Cleanup\nExit") -> (w273:string)
        n114 = call "Enqueue Multiple States.vi"("State(s) at Front"=w273, "queue in"=w276) -> ()  [unwired: 13 in, 1 out]
      }
      frame "---------- Timer ----------" {
        # "Template Separator\n(You can make a copy of, or modify, this frame)"
        n115 = call "Enqueue Multiple States.vi"("queue in"=w282) -> ()  [unwired: 14 in, 1 out]
      }
      frame "Timer: Reset" {
        n116 = call "Timer FGV.vi"("Mode"=FGV_Actions."Write", "error in (no error)"=w288, "Timer Value (s)"=5.0) -> ("error out"=w287:errorcluster)  [unwired: 6 in, 2 out]
      }
      frame "Timer: Poll" {
        n117 = call "Timer FGV.vi"("Mode"=FGV_Actions."Read", "error in (no error)"=w297) -> ("error out"=w296:errorcluster, "Expired?"=w294:bool)  [unwired: 7 in, 1 out]
        n118 = Select(t="Data: Save Hotkey\nData: Get Hotkeys", s=w294, f="UI: Listen") -> (s? t:f=w290:string)
        n119 = call "Enqueue Multiple States.vi"("queue in"=w291, "State(s) at Back"=w290) -> ()  [unwired: 13 in, 1 out]
      }
    }
  }
  n120 = Merge Errors(w9, w8) -> (w10:errorcluster)
  n121 = Release Queue(queue=w11, error in (no error)=w10) -> (error out=→"error out":errorcluster)  [unwired: 1 in, 2 out]
